vi "Delete from array if length.vi"(9 "Begin Length In":i32, 11 "Int Array In":i32[](array[numeric])) -> (3 "Int Array Out":i32[](array[numeric]))   [LabVIEW 2024]
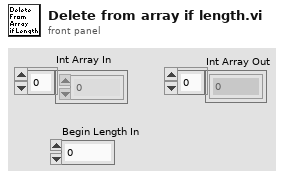
[diagram p1: front panel]
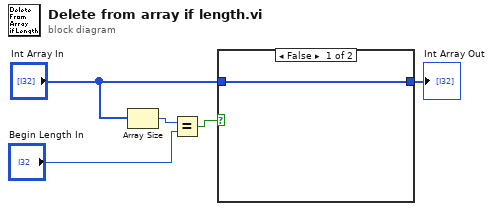
[diagram p0: block diagram]
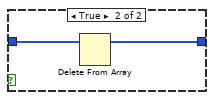
[diagram p2: hidden frame]
diagram:
  n1 = Array Size(array="Int Array In") -> (size(s)=w3:i32)
  n2 = Equal?(x=w3, y="Begin Length In") -> (x = y?=w4:bool)
  n3 = case shown="False" w4 {
    tunnel: "Int Array In" -> [w6 w8]
    tunnel: [w6 w7] -> w1
    frame False {
    }
    frame True {
      n4 = Delete From Array(array=w8) -> (array with subset deleted=w7:i32[])  [unwired: 2 in, 1 out]
    }
  }
  "Int Array Out" <- w1
